vi "target.vi"   [LabVIEW 2020]
uses:
  <vilib>/rvi/interface/RandomDataEmulation/niFpgaRandomDataHandleErrors.vi
  matrix_vector_multiply_VIs/10_5_matrix_vector_multiply.vi
  <vilib>/rvi/DataTransferAndStorage/Container/XNode/niFpgaContainer.xnode
  <vilib>/rvi/interface/RandomDataEmulation/nirviRandomDataFpgaReadWriteTemplate.vi
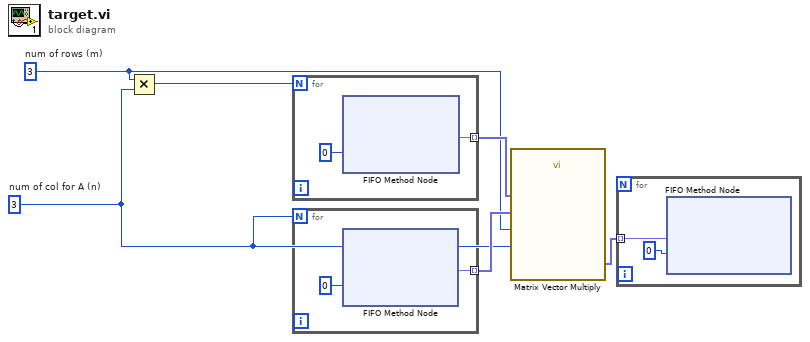
[diagram p0: block diagram]
diagram:
  w1 = 3  # num of col for A (n)
  w3 = 3  # num of rows (m)
  n1 = Multiply(x=w3, y=w1) -> (x*y=w6:i32)
  n2 = for {
    N: w6 -> [_]
    tunnel: [w8] -> w5 mode=indexing
    n3 = xnode ("FIFO Method Node")("Timeout"=0) -> ("Element"=w8:fxp<+/-,10,5>)  [unwired: 1 in, 2 out]
  }
  n4 = for {
    N: w1 -> [_]
    tunnel: [w9] -> w4 mode=indexing
    n5 = xnode ("FIFO Method Node")("Timeout"=0) -> ("Element"=w9:fxp<+/-,10,5>)  [unwired: 1 in, 2 out]
  }
  n6 = call-poly "Matrix Vector Multiply.vi"("n"=w1, "m"=w3, "B"=w4, "A"=w5) -> ("C"=w2:fxp<+/-,10,5>[])  [unwired: 2 in]
  n7 = for {
    tunnel: w2 -> [w12] mode=indexing
    n8 = xnode ("FIFO Method Node")("Element"=w12, "Timeout"=0) -> ()  [unwired: 1 in, 2 out]
  }
